vi "Transmit Data from File.vi"() -> ()   [LabVIEW 2019]
doc: "The example program opens the specified card and core, and configures the \ntransmit channel with an asynchronous transmit list buffer. The program reads \na data file and transmits that data with the specified label."
uses:
  <instrlib>/BTI429Lib/Public/Controls/429 Message List Status.ctl
  <instrlib>/BTICardLib/Private/Initialize By Card Number and Core Number.vi
  <instrlib>/BTICardLib/Private/Configure Core From XML.vi
  <instrlib>/BTI429Lib/Private/Tx/Configure/Configure Tx Channel From XML.vi
  <instrlib>/BTI429Lib/Private/Core/Action-Status/Start Channel.vi
  <instrlib>/BTI429Lib/Private/Tx/Data/Transmit Message Dynamic.vi
  <instrlib>/BTI429Lib/Private/Core/Action-Status/Stop Channel.vi
  <instrlib>/BTICardLib/BTICardLV.lvlib
  <instrlib>/BTI429Lib/BTI429LV.lvlib
panel:
  out "channel number":i32
  out "core number":i32
  out "Current Data":u32 format="%08x"
  in  "Label":u32=83 format="%o"
  in  "stop":bool
  out "error out":errorcluster
  in  "Data File":string="Data File.dat"
  in  "Channel XML Configuration File":string="Channel Config.xml"
  in  "Core XML Configuration File":string="Core Config.xml"
  in  "Card Number":i32
  # "ARINC 429: Transmit Data From File"
  # "©2016 Astronics Ballard Technology"
  # "The example program opens the specified card and core, and configures the \ntransmit channel with an asynchronous transmit list buffer. The program reads \na data file and transmits that data with the specified label."
  # "Always Stop the card\nand Close the card when\ndone. Otherwise, the hardware\ncontinues to operate."
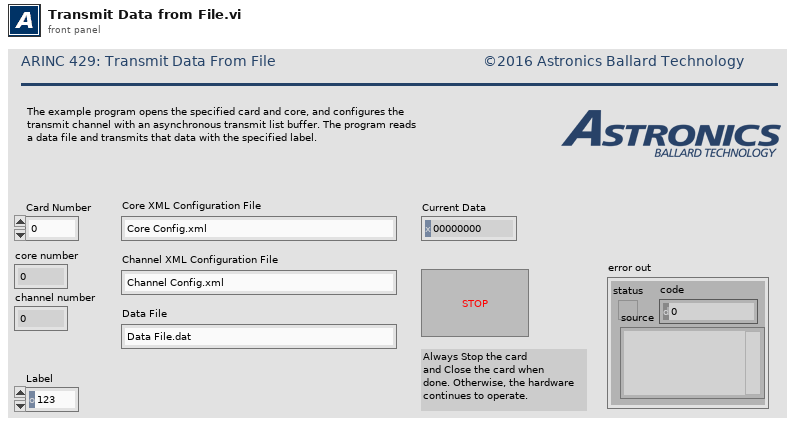
[diagram p1: front panel]
types:
  T1 = typedef "BTI429LV.lvlib/429 Message List Status.ctl" = u32
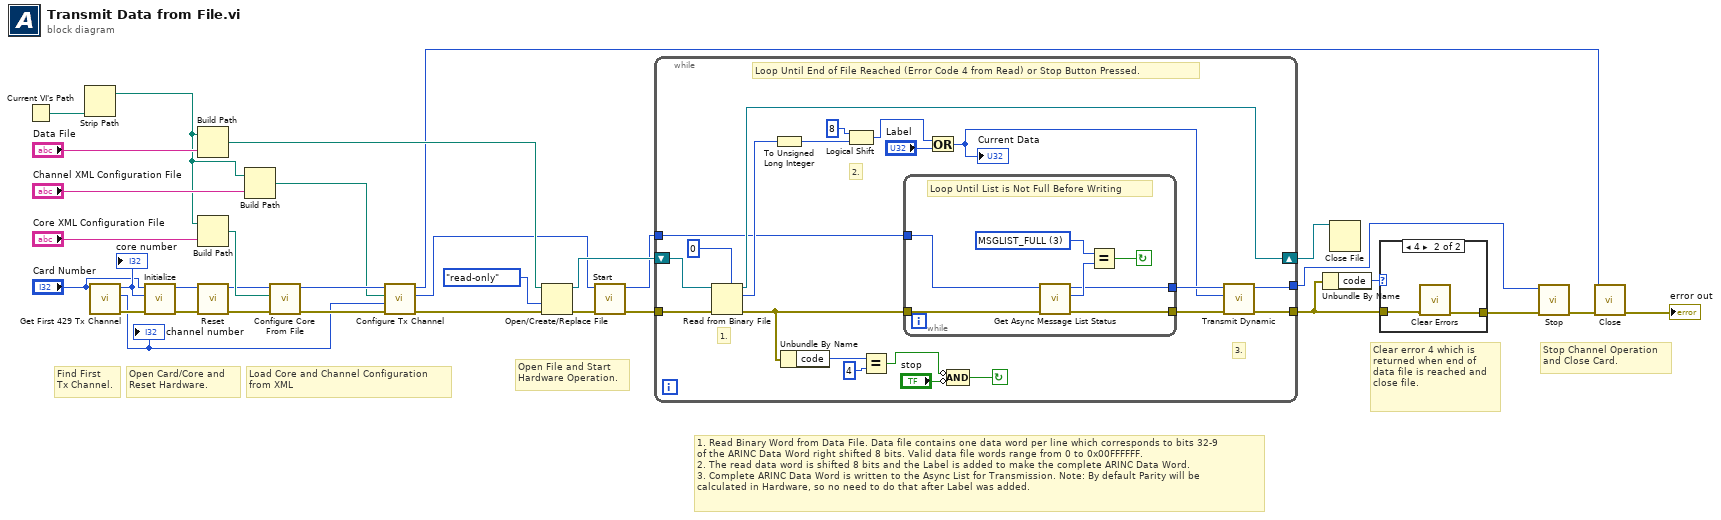
[diagram p0: block diagram]
diagram:
  # "Find First\nTx Channel."
  # "Open File and Start\nHardware Operation."
  # "Load Core and Channel Configuration\nfrom XML"
  # "Open Card/Core and\nReset Hardware."
  # "Stop Channel Operation\nand Close Card."
  # "1. Read Binary Word from Data File. Data file contains one data word per line which corresponds to bits 32-9\nof the ARINC Data Word right shifted 8 bits. Valid data file words range from 0 to 0x00FFFFFF.\n2. The read data word is shifted 8 bits and the Label is added to make the complete ARINC Data Word.\n3. Complete ARINC Data Word is written to the Async List for Transmission. Note: By default Parity will be\ncalculated in Hardware, so no need to do that after Label was added."
  # "Clear error 4 which is returned when end of data file is reached and close file."
  n1 = Current VI's Path() -> (path=w25:path)
  n2 = Strip Path(path=w25) -> (stripped path=w18:path)  [unwired: 1 out]
  n3 = call "Get First 429 Tx Channel.vi"("Card Number"="Card Number") -> ("error out"=w6:errorcluster, "Channel Number"=w5:i32, "Core Number"=w8:i32)  [unwired: 8 in]
  "core number" <- w8
  "channel number" <- w5
  n4 = call-poly <instrlib>:"Initialize.vi"("error in (no error)"=w6, "core number"=w8, "card number"="Card Number") -> ("error out"=w10:errorcluster, "core handle out"=w12:u64)  [unwired: 7 in]
  n5 = Build Path(base path=w18, name or relative path="Data File") -> (appended path=w17:path)
  n6 = Build Path(base path=w18, name or relative path="Core XML Configuration File") -> (appended path=w23:path)
  n7 = call <instrlib>:"Reset.vi"("error in (no error)"=w10, "core handle in"=w12) -> ("error out"=w9:errorcluster, "core handle out"=w11:u64)  [unwired: 8 in]
  n8 = Build Path(base path=w18, name or relative path="Channel XML Configuration File") -> (appended path=w21:path)
  n9 = call-poly <instrlib>:"Configure Core From File.vi"("error in (no error)"=w9, "configuration file path"=w23, "core handle in"=w11) -> ("error out"=w31:errorcluster, "core handle out"=w32:u64)  [unwired: 7 in]
  n10 = call-poly <instrlib>:"Configure Tx Channel.vi"("error in (no error)"=w31, "channel number in"=w5, "configuration file path"=w21, "core handle in"=w32) -> ("error out"=w20:errorcluster, "channel handle out"=w16:u64, "core handle out"=w14:u64)  [unwired: 5 in]
  n11 = Open/Create/Replace File(file path (use dialog)=w17, error in=w20, access (0:read/write)=enum16{"read/write", "read-only", "write-only"}."read-only") -> (refnum out=w29:refnum<file>, error out=w28:errorcluster)  [unwired: 3 in, 1 out]
  n12 = call-poly <instrlib>:"Start.vi"("error in (no error)"=w28, "channel handle in"=w16) -> ("error out"=w27:errorcluster, "channel handle out"=w15:u64)  [unwired: 8 in]
  n13 = while {
    tunnel: w27 -> [w51]
    shift-right: [w49] -> w13
    shift-left: w29 -> [w54]
    tunnel: [w41] -> w2
    tunnel: w15 -> [w38]
    tunnel: [w44] -> w1
    stop <- w53 continue-if-true
    # "3."
    # "2."
    # "1."
    # "Loop Until End of File Reached (Error Code 4 from Read) or Stop Button Pressed."
    n14 = Read from Binary File(5:u16 0, 8:w51, 11:w54) -> (0:w34:errorcluster, 2:w48:u16, 3:w49:refnum<file>)  [unwired: 3 in, 1 out]
    n15 = To Unsigned Long Integer(number=w48) -> (unsigned 32bit integer=w47:u32)
    n16 = Unbundle By Name(w34) -> ("code"=w42:i32)
    n17 = Logical Shift(y=8, x=w47) -> (x << y=w39:u32)
    n18 = Equal?(x=w42, y=4) -> (x = y?=w40:bool)
    n19 = while {
      tunnel: w34 -> [w58]
      tunnel: [w57] -> w35
      tunnel: w38 -> [w56]
      tunnel: [w55] -> w37
      stop <- w59 continue-if-true
      w60 = T1 3 items=["MSGLIST_INVALID", "MSGLIST_EMPTY", "MSGLIST_PARTIAL", "MSGLIST_FULL", "MSGLIST_OFF"] ("list status out")
      # "Loop Until List is Not Full Before Writing"
      n20 = call <instrlib>:"Get Async Message List Status.vi"("error in (no error)"=w58, "channel handle in"=w56) -> ("error out"=w57:errorcluster, "list status out"=w61:T1, "channel handle out"=w55:u64)  [unwired: 7 in]
      n21 = Equal?(x=w60, y=w61) -> (x = y?=w59:bool)
    }
    n22 = Or(x=w39, y="Label") -> (x .or. y?=w36:u32)
    "Current Data" <- w36
    n23 = Compound Arithmetic op=AND(invert w40, invert "stop") -> (w53:bool)
    n24 = call-poly <instrlib>:"Transmit Dynamic.vi"("error in (no error)"=w35, "message data"=w36, "channel handle in"=w37) -> ("error out"=w41:errorcluster, "channel handle out"=w44:u64)  [unwired: 7 in]
  }
  n25 = Unbundle By Name(w2) -> ("code"=w4:i32)
  n26 = Close File(refnum=w13) -> ()  [unwired: 1 in, 2 out]
  n27 = case shown="4" w4 {
    tunnel: [w62 w64] -> w3
    tunnel: w2 -> [w62 w63]
    frame Default {
    }
    frame 4 {
      n28 = call <vilib>:"Clear Errors.vi"("error in (no error)"=w63) -> ("error out"=w64:errorcluster)  [unwired: 5 in, 1 out]
    }
  }
  n29 = call-poly <instrlib>:"Stop.vi"("error in (no error)"=w3, "channel handle in"=w1) -> ("error out"=w33:errorcluster)  [unwired: 8 in, 1 out]
  n30 = call <instrlib>:"Close.vi"("error in (no error)"=w33, "core handle in"=w14) -> ("error out"=→"error out":errorcluster)  [unwired: 8 in, 1 out]
